vi "Insert Dynamic Size Panels.vi"(8 "error in (no error)":errorcluster, 11 "PanelArray in":refnum<class "PanelArray.lvclass">) -> (0 "error out":errorcluster, 3 "PanelArray out":refnum<class "PanelArray.lvclass">)   [LabVIEW 2018, in "OOPanel.lvlib" / "PanelArray.lvclass"]
uses:
  PanelArray.lvclass
  PanelArray.lvclass/PanelArray.ctl
  Panel/State.ctl
  Panel/Panel.lvclass
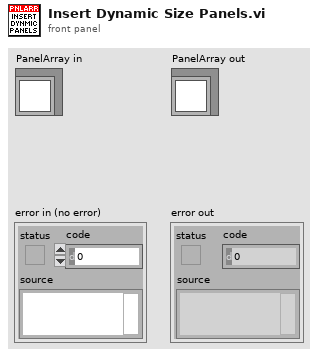
[diagram p1: front panel]
types:
  T1 = typedef "OOPanel.lvlib/PanelArray.lvclass/Ref Data.ctl" = cluster{"State":T2, "Refs":T3, "Events":T4, "Scrolling":T5, "Panels":T6}
  T2 = typedef "OOPanel.lvlib/PanelArray.lvclass/State.ctl" = cluster{"Defer Updates":bool, "Running":bool, "Dynamic Sizing":bool, "Borders":bool}
  T3 = typedef "OOPanel.lvlib/PanelArray.lvclass/Refs.ctl" = cluster{"SubPanels":refnum<vi>[], "Scrollbar":refnum<vi>, "Owning Panel":refnum<vi>}
  T4 = typedef "OOPanel.lvlib/PanelArray.lvclass/Events.ctl" = cluster{"Close":refnum<user-event>}
  T5 = typedef "OOPanel.lvlib/PanelArray.lvclass/Scrolling.ctl" = cluster{"Size":i32, "Max":i32, "Current":i32, "Top Index":i32, "Heights":i32[]}
  T6 = typedef "OOPanel.lvlib/PanelArray.lvclass/Panels.ctl" = cluster{"All":refnum<class "Panel.lvclass">[], "Visible":refnum<class "Panel.lvclass">[], "Blank":refnum<class "ArrayBlank.lvclass">}
  T7 = typedef "OOPanel.lvlib/Panel.lvclass/State.ctl" = enum16{"Idle", "Hidden", "Visible", "Subpanel"}
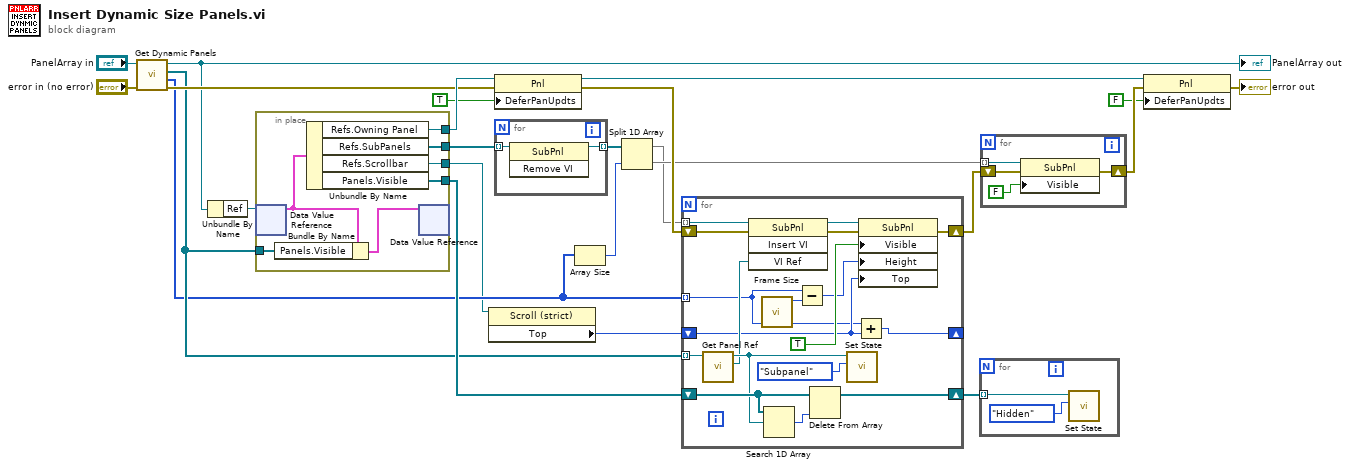
[diagram p0: block diagram]
diagram:
  n1 = call "Get Dynamic Panels.vi"("error in (no error)"="error in (no error)", "PanelArray in"="PanelArray in") -> ("error out"=w9:errorcluster, "Heights"=w2:i32[], "Visible Panels"=w6:refnum<class "Panel.lvclass">[], "PanelArray out"=w8:refnum<class "PanelArray.lvclass">)  [unwired: 6 in]
  "PanelArray out" <- w8
  n2 = Unbundle By Name(w8) -> ("Ref"=w24:refnum<data-value>)
  n3 = in-place {
    in-place-border: [w31] -> w3
    in-place-border: w6 -> [w28]
    in-place-border: [w27] -> w22
    in-place-border: [w26] -> w16
    in-place-border: [w25] -> w1
    n4 = in-place-dvr #1(w24) -> (w30:T1)  [unwired: 1 out]
    n5 = Bundle By Name(cluster=w30, "Panels.Visible"=w28) -> (w29:T1)
    n6 = Unbundle By Name(w30) -> ("Refs.Owning Panel"=w27:refnum<vi>, "Refs.SubPanels"=w31:refnum<vi>[], "Refs.Scrollbar"=w25:refnum<vi>, "Panels.Visible"=w26:refnum<class "Panel.lvclass">[])
    n7 = in-place-dvr #1(w29) -> ()  [unwired: 2 out]
  }
  n8 = property class="Scroll (strict)"(reference=w1) -> ("Top"=w4:i32)  [unwired: 1 in, 2 out]
  n9 = property class="Pnl"(reference=w22, error in=w9, "DeferPanUpdts"=TRUE ("Defer Panel Updates")) -> (reference out=w11:refnum<vi>, error out=w20:errorcluster)
  n10 = for {
    tunnel: w3 -> [w33] mode=indexing
    tunnel: [w32] -> w19 mode=indexing
    n11 = invoke class="SubPnl" method="Remove VI"(reference=w33) -> (reference out=w32:refnum<vi>)  [unwired: 2 in, 2 out]
  }
  n12 = Array Size(array=w2) -> (size(s)=w23:i32)
  n13 = Split 1D Array(array=w19, index=w23) -> (first subarray=w5:refnum<vi>[], second subarray=w18:refnum<vi>[])
  n14 = for {
    tunnel: w6 -> [w51] mode=indexing
    tunnel: w5 -> [w50] mode=indexing
    shift-right: [w38] -> w17
    shift-left: w20 -> [w49]
    shift-right: [w44] -> w15
    shift-left: w16 -> [w46]
    tunnel: w2 -> [w36] mode=indexing
    shift-right: [w39] -> _
    shift-left: w4 -> [w40]
    n15 = call "Get Panel Ref.vi"("Panel in"=w51) -> ("Panel Ref"=w41:refnum<vi>, "Panel out"=w42:refnum<class "Panel.lvclass">)  [unwired: 8 in, 1 out]
    n16 = invoke class="SubPnl" method="Insert VI"(reference=w50, error in=w49, "VI Ref"=w41) -> (reference out=w48:refnum<vi>, error out=w47:errorcluster)  [unwired: 1 in, 2 out]
    n17 = call "Frame Size.vi"() -> ("Frame Size"=w37:i32)  [unwired: 11 in]
    n18 = Search 1D Array(1D array=w46, element=w42) -> (index of element=w45:i32)  [unwired: 1 in]
    n19 = Subtract(x=w36, y=w37) -> (x-y=w35:i32)
    n20 = Delete From Array(array=w46, index=w45) -> (array with subset deleted=w44:refnum<class "Panel.lvclass">[])  [unwired: 1 in, 1 out]
    n21 = call "Set State.vi"("State"=State."Subpanel", "Panel in"=w42) -> ()  [unwired: 8 in, 2 out]
    n22 = Add(x=w36, y=w40) -> (x+y=w39:i32)
    n23 = property class="SubPnl"(reference=w48, error in=w47, "Visible"=TRUE, "Height"=w35, "Top"=w40) -> (error out=w38:errorcluster)  [unwired: 1 out]
  }
  n24 = for {
    tunnel: w15 -> [w52] mode=indexing
    n25 = call "Set State.vi"("State"=State."Hidden", "Panel in"=w52) -> ()  [unwired: 8 in, 2 out]
  }
  n26 = for {
    tunnel: w18 -> [w57] mode=indexing
    shift-right: [w54] -> w14
    shift-left: w17 -> [w56]
    n27 = property class="SubPnl"(reference=w57, error in=w56, "Visible"=FALSE) -> (error out=w54:errorcluster)  [unwired: 1 out]
  }
  n28 = property class="Pnl"(reference=w11, error in=w14, "DeferPanUpdts"=FALSE ("Defer Panel Updates")) -> (error out=→"error out":errorcluster)  [unwired: 1 out]
